vi "NI VeriStand - Create Section.vi"(8 "Error in":errorcluster, 10 "GUID":string="03D3BB89-1485-13A6-56005DE6430FF8B7", 11 "Section Name":string="InportSection") -> (0 "Error out":errorcluster, 3 "NodeID":u64)   [LabVIEW 2025, in "NI_VS RuntimeConfigurationFile ScriptingAPI.lvlib"]
uses:
  NI_VS RuntimeConfigurationFile ScriptingAPI.lvlib
  NationalInstruments.VeriStand.SystemDefinitionAPI
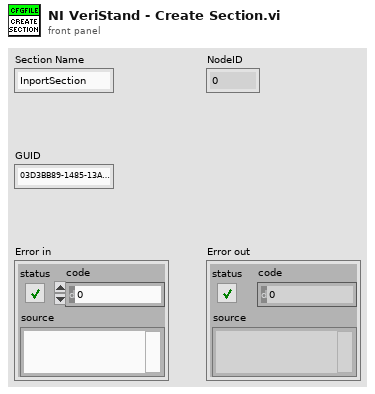
[diagram p1: front panel]
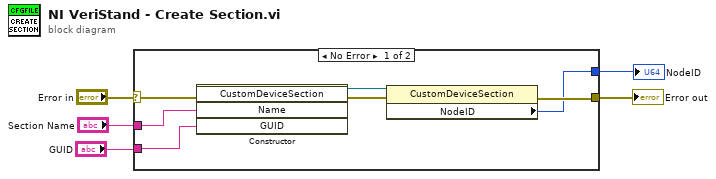
[diagram p0: block diagram]
diagram:
  n1 = case shown="No Error" "Error in" {
    selector: "Error in" -> [w12 w13]
    tunnel: [w10 w13] -> w5
    tunnel: "Section Name" -> [w9 _]
    tunnel: "GUID" -> [w8 _]
    tunnel: [w6 _] -> w1
    frame No Error {
      n2 = constructor class="CustomDeviceSection"(error in=w12, "Name"=w9, "GUID"=w8) -> (reference out=w7:refnum<k24>, error out=w11:errorcluster)  [unwired: 2 in, 3 out]
      n3 = property class="CustomDeviceSection"(reference=w7, error in=w11) -> (error out=w10:errorcluster, "NodeID"=w6:u64)  [unwired: 1 out]
    }
    frame Error {
    }
  }
  "Error out" <- w5
  "NodeID" <- w1
